vi "ManageScript.vi"(8 "Error In":errorcluster) -> (0 "Error Out":errorcluster)   [LabVIEW 2018]
doc: "This VI allows the user to edit, view, and create new script."
uses:
  <vilib>/Utility/config.llb/NI_LVConfig.lvlib
panel:
  in  "Save As":bool
  out "Array 4":bool[](array[boolean])
  out "Array 3":string[](array[string])
  out "Array 2":path[](array[path])
  out "Array":string[][](array[string])
  out "Numeric Control":i32
  in  "Script Names":string[](array[string])
  in  "Script Locations":path[](array[path])
  in  "Tab Control":enum32{"Edit Script", "View Script"}(tab)
  in  "Script to Edit":string[](array[string])
  in  "Read":bool
  out "Script to View":string
  in  "Close Button":bool
  in  "Save Button":bool
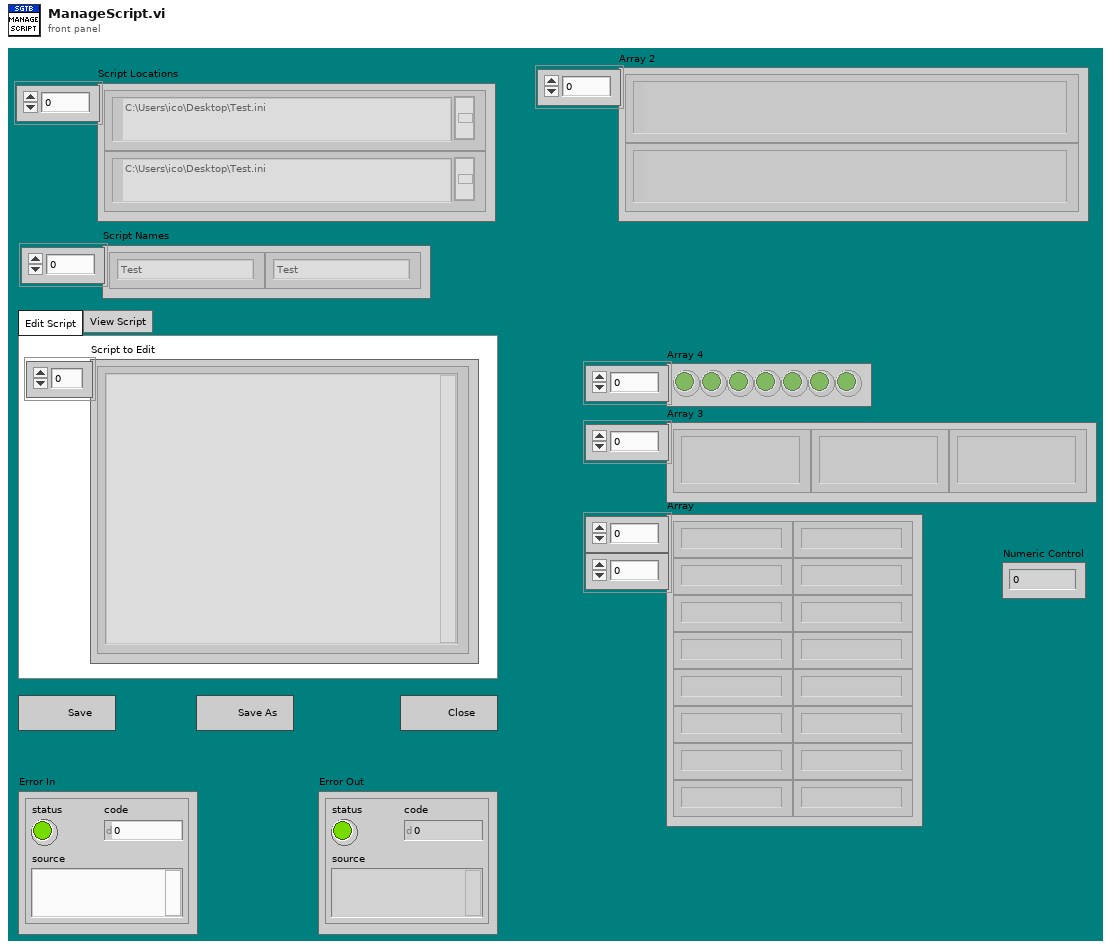
[diagram p1: front panel]
types:
  T1 = enum32{"Invalid", "Standard", "Closed", "Hidden", "Minimized", "Maximized"}
  T2 = enum32{"Invalid", "Default", "Floating", "Floating/Auto-Hide", "Modal"}
  T3 = typedef "NI_LVConfig.lvlib/Config Data RefNum.ctl" = refnum<k1>
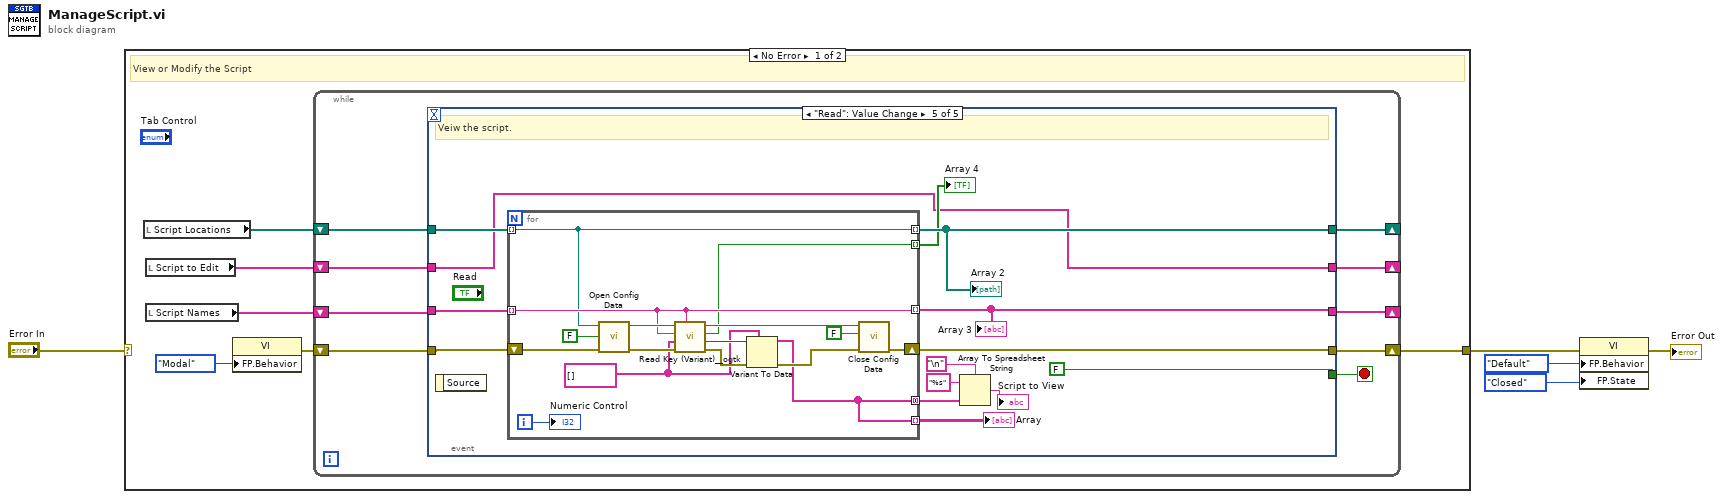
[diagram p0: block diagram]
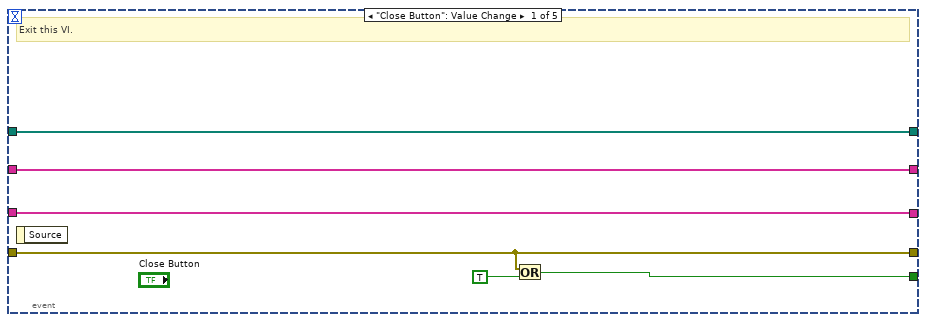
[diagram p2: hidden frame]
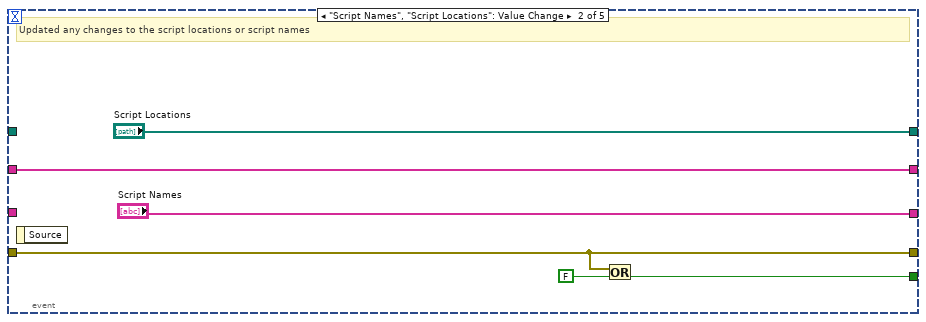
[diagram p3: hidden frame]
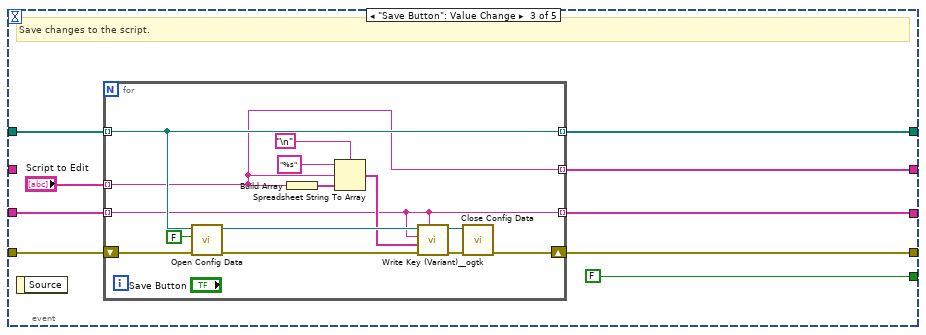
[diagram p4: hidden frame]
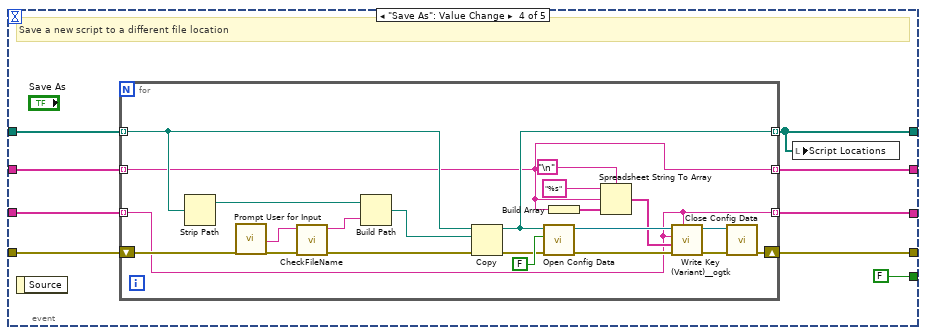
[diagram p5: hidden frame]
diagram:
  n1 = case shown="No Error" "Error In" {
    selector: "Error In" -> [_ w117]
    tunnel: [w6 w117] -> w3
    frame No Error {
      # "View or Modify the Script"
      n2 = local read "Script Locations"() -> (w8:path[])
      n3 = local read "Script to Edit"() -> (w7:string[])
      n4 = local read "Script Names"() -> (w9:string[])
      n5 = property class="VI"("FP.Behavior"=T2."Modal" ("Front Panel Window:Behavior")) -> (error out=w11:errorcluster)  [unwired: 2 in, 1 out]
      n6 = while {
        shift-right: [w18] -> w6
        shift-left: w11 -> [w19]
        shift-right: [w16] -> _
        shift-left: w8 -> [w17]
        shift-right: [w14] -> _
        shift-left: w9 -> [w15]
        shift-right: [w12] -> _
        shift-left: w7 -> [w13]
        stop <- w20 stop-if-true
        n7 = event shown="[4] \"Read\": Value Change" {
          selector: _ -> [_ _ _ _ _]
          dyn-events: _ -> [_ _ _ _ _]
          timeout: _ -> [_ _ _ _ _]
          tunnel: [w25 w29 FALSE FALSE FALSE] -> w20
          tunnel: w17 -> [w23 _ w40 w63 w98]
          tunnel: w15 -> [w22 _ w38 w62 w97]
          tunnel: w19 -> [w24 w28 w41 w64 w100]
          tunnel: [w24 w28 w36 w61 w99] -> w18
          tunnel: [w23 "Script Locations" w37 w56 w91] -> w16
          tunnel: [w22 "Script Names" w34 w59 w96] -> w14
          tunnel: w13 -> [w21 w27 _ w58 w87]
          tunnel: [w21 w27 w33 w57 w87] -> w12
          event "Close Button": Value Change {
            # "Exit this VI."
            n8 = event-data() -> ()  [unwired: 1 in, 1 out]
            n9 = Or(x=w24, y=TRUE) -> (x .or. y?=w25:bool)
          }
          event "Script Names", "Script Locations": Value Change {
            # "Updated any changes to the script locations or script names"
            n10 = event-data() -> ()  [unwired: 1 in, 1 out]
            n11 = Or(x=w28, y=FALSE) -> (x .or. y?=w29:bool)
          }
          event "Save Button": Value Change {
            # "Save changes to the script."
            n12 = event-data() -> ()  [unwired: 1 in, 1 out]
            n13 = for {
              shift-right: [w49] -> w36
              shift-left: w41 -> [w50]
              tunnel: w40 -> [w44] mode=indexing
              tunnel: "Script to Edit" -> [w42] mode=indexing
              tunnel: w38 -> [w43] mode=indexing
              tunnel: [w44] -> w37 mode=indexing
              tunnel: [w43] -> w34 mode=indexing
              tunnel: [w42] -> w33 mode=indexing
              n14 = call <vilib>:"Open Config Data.vi"("error in (no error)"=w50, "create file if necessary (T)"=FALSE, "configuration file path"=w44) -> ("error out"=w54:errorcluster, "refnum"=w52:T3)  [unwired: 6 in, 1 out]
              n15 = Build Array(w42) -> (w48:string[])
              n16 = Spreadsheet String To Array(delimiter (Tab)="\n", format string="%s", spreadsheet string=w42, array type (2D Dbl)=w48) -> (array=w45:string[])
              n17 = call <userlib>:"Write Key (Variant)__ogtk.vi"("section"=w43, "error in (no error)"=w54, "key-value"=w45, "key (optional)"=w43, "refnum"=w52) -> ("error out"=w53:errorcluster, "refnum out"=w51:T3)  [unwired: 5 in]
              n18 = call <vilib>:"Close Config Data.vi"("error in (no error)"=w53, "refnum"=w51) -> ("error out"=w49:errorcluster)  [unwired: 8 in, 1 out]
            }
          }
          event "Save As": Value Change {
            # "Save a new script to a different file location"
            n19 = event-data() -> ()  [unwired: 1 in, 1 out]
            n20 = for {
              shift-right: [w81] -> w61
              shift-left: w64 -> [w70]
              tunnel: w63 -> [w69] mode=indexing
              tunnel: w58 -> [w65] mode=indexing
              tunnel: w62 -> [w66] mode=indexing
              tunnel: [w68] -> w56 mode=indexing
              tunnel: [w66] -> w59 mode=indexing
              tunnel: [w65] -> w57 mode=indexing
              n21 = Strip Path(path=w69) -> (stripped path=w72:path)  [unwired: 1 out]
              n22 = call "Prompt User for Input"("error in (no error)"=w70) -> ("File Name"=w67:string, "error out"=w74:errorcluster)  [unwired: 16 in, 1 out]
              n23 = call "CheckFileName.vi"("Error In"=w74, "File Name in"=w67) -> ("Error Out"=w75:errorcluster, "File Name out"=w76:string)  [unwired: 8 in]
              n24 = Build Path(base path=w72, name or relative path=w76) -> (appended path=w73:path)
              n25 = Copy(8:w75, 10:w73, 11:w69) -> (0:w71:errorcluster, 3:w68:path)  [unwired: 2 in, 1 out]
              n26 = call <vilib>:"Open Config Data.vi"("error in (no error)"=w71, "create file if necessary (T)"=FALSE, "configuration file path"=w68) -> ("error out"=w85:errorcluster, "refnum"=w83:T3)  [unwired: 6 in, 1 out]
              n27 = Build Array(w65) -> (w80:string[])
              n28 = Spreadsheet String To Array(delimiter (Tab)="\n", format string="%s", spreadsheet string=w65, array type (2D Dbl)=w80) -> (array=w77:string[])
              n29 = call <userlib>:"Write Key (Variant)__ogtk.vi"("section"=w66, "error in (no error)"=w85, "key-value"=w77, "key (optional)"=w66, "refnum"=w83) -> ("error out"=w84:errorcluster, "refnum out"=w82:T3)  [unwired: 5 in]
              n30 = call <vilib>:"Close Config Data.vi"("error in (no error)"=w84, "refnum"=w82) -> ("error out"=w81:errorcluster)  [unwired: 8 in, 1 out]
            }
            n31 = local write "Script Locations"(w56) -> ()
          }
          event "Read": Value Change {
            # "Veiw the script."
            n32 = event-data() -> ()  [unwired: 1 in, 1 out]
            n33 = for {
              tunnel: w98 -> [w105] mode=indexing
              tunnel: w97 -> [w106] mode=indexing
              shift-right: [w114] -> w99
              shift-left: w100 -> [w115]
              tunnel: [w106] -> w96 mode=indexing
              tunnel: [w102] -> w92 mode=concatenating
              tunnel: [w105] -> w91 mode=indexing
              tunnel: [w102] -> w90 mode=indexing
              tunnel: [w101] -> w89 mode=indexing
              i -> [w103]
              w104 = string[] []
              n34 = call <vilib>:"Open Config Data.vi"("error in (no error)"=w115, "create file if necessary (T)"=FALSE, "configuration file path"=w105) -> ("error out"=w111:errorcluster, "refnum"=w109:T3)  [unwired: 6 in, 1 out]
              n35 = call <userlib>:"Read Key (Variant)__ogtk.vi"("section"=w106, "error in (no error)"=w111, "type"=w104, "key (optional)"=w106, "refnum"=w109) -> ("error out"=w112:errorcluster, "key-value"=w113:variant, "found?"=w101:bool, "refnum out"=w108:T3)  [unwired: 3 in]
              n36 = Variant To Data(error in=w112, type=w104, Variant=w113) -> (data=w102:string[], error out=w110:errorcluster)
              n37 = call <vilib>:"Close Config Data.vi"("error in (no error)"=w110, "write file if changed (T)"=FALSE, "refnum"=w108) -> ("error out"=w114:errorcluster)  [unwired: 7 in, 1 out]
              "Numeric Control" <- w103
            }
            "Array" <- w90
            "Array 2" <- w91
            "Array 3" <- w96
            "Array 4" <- w89
            n38 = Array To Spreadsheet String(delimiter (Tab)="\n", array=w92, 3:"%s" ("format string")) -> (spreadsheet string=→"Script to View":string)
          }
        }
      }
    }
    frame Error {
    }
  }
  n39 = property class="VI"(error in=w3, "FP.Behavior"=T2."Default" ("Front Panel Window:Behavior"), "FP.State"=T1."Closed" ("Front Panel Window:State")) -> (error out=→"Error Out":errorcluster)  [unwired: 1 in, 1 out]
